vi "GPS NMEA Main Processor (SubVI).vi"(11 "GPS Buffer In":string) -> (1 "output cluster":T1, 2 "'\\n' not found?":bool, 3 "GPS Buffer Out":string)   [LabVIEW 2015]
doc: "NMEA data string parser"
panel:
  out "Date":string
  out "Time":string
  out "Latitude":string
  out "Longitude":string
  out "Alt (m)":string
  out "Speed (knots)":string
  out "Array of Strings":string[](array[string])
  out "work string":string
  out "broken string":string
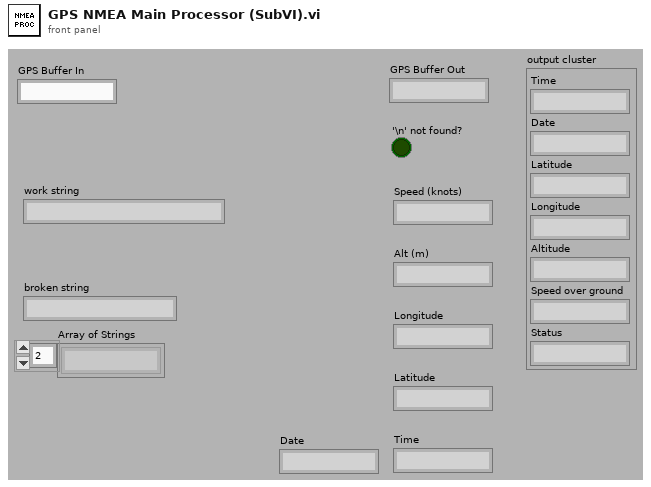
[diagram p1: front panel]
types:
  T1 = cluster{"Time":string, "Date":string, "Latitude":string, "Longitude":string, "Altitude":string, "Speed over ground":string, "Status":string}
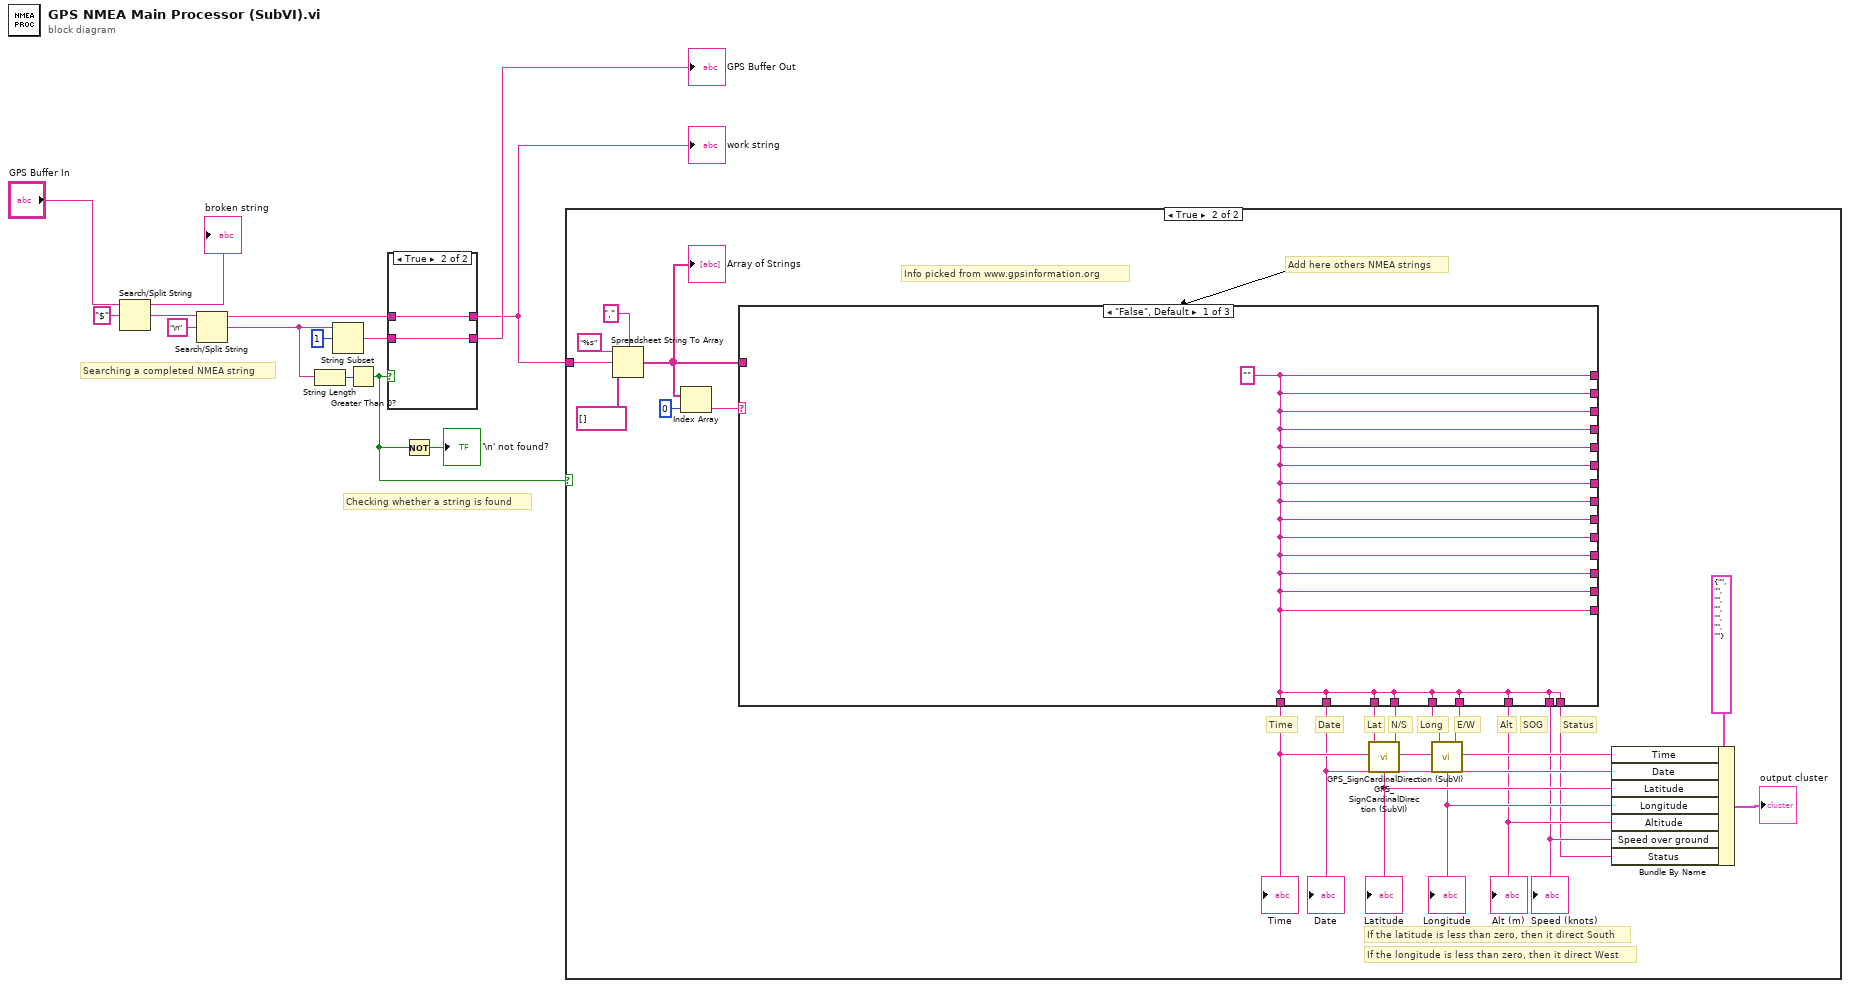
[diagram p0: block diagram]
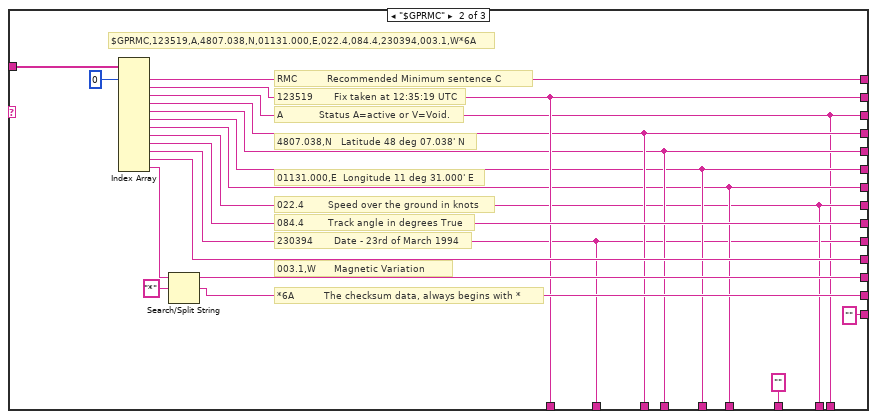
[diagram p3: hidden frame]
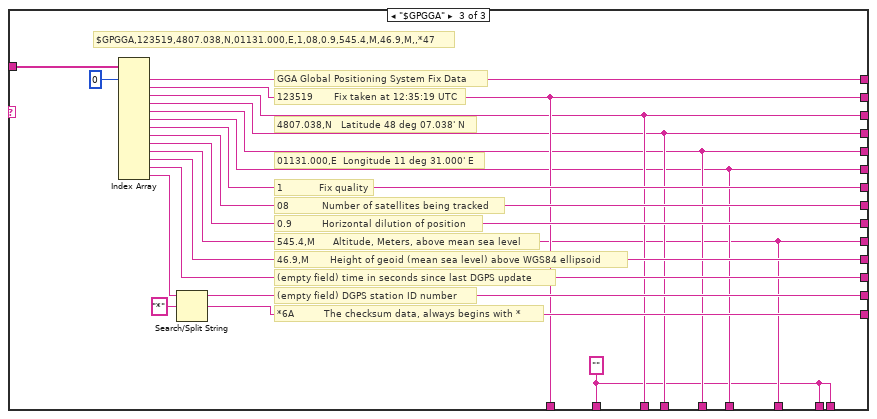
[diagram p4: hidden frame]
diagram:
  # "Checking whether a string is found"
  # "Searching a completed NMEA string"
  n1 = Search/Split String(string="GPS Buffer In", search string/char (-)="$") -> (substring before match=→"broken string":string, match + rest of string=w12:string)  [unwired: 1 in, 1 out]
  n2 = Search/Split String(string=w12, search string/char (-)="\n") -> (substring before match=w8:string, match + rest of string=w5:string)  [unwired: 1 in, 1 out]
  n3 = String Length(string=w5) -> (length=w4:i32)
  n4 = String Subset(string=w5, offset (0)=1) -> (substring=w7:string)  [unwired: 1 in]
  n5 = Greater Than 0?(x=w4) -> (x > 0?=w1:bool)
  n6 = case shown="True" w1 {
    tunnel: w8 -> [w15 w18]
    tunnel: [w16 w18] -> w3
    tunnel: w7 -> [w16 w17]
    tunnel: [w15 w17] -> w6
    frame False {
    }
    frame True {
    }
  }
  "work string" <- w3
  "GPS Buffer Out" <- w6
  n7 = Not(x=w1) -> (.not. x?=→"'\\n' not found?":bool)
  n8 = case shown="True" w1 {
    tunnel: w3 -> [_ w28]
    frame False {
    }
    frame True {
      # "Add here others NMEA strings"
      # "Status"
      # "If the longitude is less than zero, then it direct West"
      # "If the latitude is less than zero, then it direct South"
      # "Date"
      # "SOG"
      # "Alt"
      # "E/W"
      # "Long"
      # "N/S"
      # "Lat"
      # "Time"
      # "Info picked from www.gpsinformation.org"
      n9 = Spreadsheet String To Array(delimiter (Tab)=",", format string="%s", spreadsheet string=w28, array type (2D Dbl)=string[] [] ("Array Constant")) -> (array=w29:string[])
      "Array of Strings" <- w29
      n10 = Index Array(array=w29, index=0) -> (element=w33:string)
      n11 = case shown="\"False\", Default" w33 {
        tunnel: w29 -> [_ w58 w77]
        tunnel: [w39 w56 w75] -> _
        tunnel: [w39 w48 w65] -> _
        tunnel: [w39 w40 w64] -> _
        tunnel: [w39 w47 w63] -> _
        tunnel: [w39 w46 w62] -> _
        tunnel: [w39 w45 w61] -> _
        tunnel: [w39 w44 w74] -> _
        tunnel: [w39 w43 w73] -> _
        tunnel: [w39 w55 w72] -> _
        tunnel: [w39 w41 w60] -> _
        tunnel: [w39 w54 w71] -> _
        tunnel: [w39 w51 w67] -> _
        tunnel: [w39 w50 w69] -> _
        tunnel: [w39 "" w66] -> _
        tunnel: [w39 w48 w65] -> w27
        tunnel: [w39 w47 w64] -> w35
        tunnel: [w39 w46 w63] -> w36
        tunnel: [w39 w45 w62] -> w37
        tunnel: [w39 w44 w61] -> w38
        tunnel: [w39 "" w60] -> w23
        tunnel: [w39 w43 w59] -> w22
        tunnel: [w39 w41 w59] -> w26
        tunnel: [w39 w40 w59] -> w20
        frame "False", Default {
          w39 = ""
        }
        frame "$GPRMC" {
          # "$GPRMC,123519,A,4807.038,N,01131.000,E,022.4,084.4,230394,003.1,W*6A"
          # "*6A          The checksum data, always begins with *"
          # "003.1,W      Magnetic Variation"
          # "230394       Date - 23rd of March 1994"
          # "084.4        Track angle in degrees True"
          # "022.4        Speed over the ground in knots"
          # "01131.000,E  Longitude 11 deg 31.000' E"
          # "4807.038,N   Latitude 48 deg 07.038' N"
          # "A            Status A=active or V=Void."
          # "123519       Fix taken at 12:35:19 UTC"
          # "RMC          Recommended Minimum sentence C"
          n12 = Index Array(array=w58, index #1=0 ("index")) -> (element #1=w56:string, element #2=w48:string, element #3=w40:string, element #4=w47:string, element #5=w46:string, element #6=w45:string, element #7=w44:string, element #8=w43:string, element #9=w55:string, element #10=w41:string, element #11=w54:string, element #12=w53:string)  [unwired: 11 in]
          n13 = Search/Split String(string=w53, search string/char (-)="*") -> (substring before match=w50:string, match + rest of string=w51:string)  [unwired: 1 in, 1 out]
        }
        frame "$GPGGA" {
          w59 = ""
          # "(empty field) DGPS station ID number"
          # "(empty field) time in seconds since last DGPS update"
          # "46.9,M       Height of geoid (mean sea level) above WGS84 ellipsoid"
          # "545.4,M      Altitude, Meters, above mean sea level"
          # "0.9          Horizontal dilution of position"
          # "08           Number of satellites being tracked"
          # "$GPGGA,123519,4807.038,N,01131.000,E,1,08,0.9,545.4,M,46.9,M,,*47"
          # "1            Fix quality"
          # "01131.000,E  Longitude 11 deg 31.000' E"
          # "*6A          The checksum data, always begins with *"
          # "4807.038,N   Latitude 48 deg 07.038' N"
          # "123519       Fix taken at 12:35:19 UTC"
          # "GGA Global Positioning System Fix Data"
          n14 = Index Array(array=w77, index #1=0 ("index")) -> (element #1=w75:string, element #2=w65:string, element #3=w64:string, element #4=w63:string, element #5=w62:string, element #6=w61:string, element #7=w74:string, element #8=w73:string, element #9=w72:string, element #10=w60:string, element #11=w71:string, element #12=w69:string, element #13=w68:string)  [unwired: 12 in]
          n15 = Search/Split String(string=w68, search string/char (-)="*") -> (substring before match=w67:string, match + rest of string=w66:string)  [unwired: 1 in, 1 out]
        }
      }
      "Speed (knots)" <- w22
      "Alt (m)" <- w23
      "Time" <- w27
      "Date" <- w26
      n16 = call "GPS_SignCardinalDirection (SubVI).vi"("Value"=w35, "Cardinal Direction"=w36) -> ("Output Value"=w25:string)
      "Latitude" <- w25
      n17 = call "GPS_SignCardinalDirection (SubVI).vi"("Value"=w37, "Cardinal Direction"=w38) -> ("Output Value"=w24:string)
      "Longitude" <- w24
      n18 = Bundle By Name(cluster=T1 {"Time"="", "Date"="", "Latitude"="", "Longitude"="", "Altitude"="", "Speed over ground"="", "Status"=""}, "Time"=w27, "Date"=w26, "Latitude"=w25, "Longitude"=w24, "Altitude"=w23, "Speed over ground"=w22, "Status"=w20) -> (→"output cluster":T1)
    }
  }
